vi "Read Browse Options.vi"(8 "error in (no error)":errorcluster, 11 "Path.lvclass in":refnum<class "Path.lvclass">) -> (0 "error out":errorcluster, 2 "BrowseOptions":T1, 3 "Path.lvclass out":refnum<class "Path.lvclass">)   [LabVIEW 2015, in "Path.lvclass"]
uses:
  Path.lvclass
  <vilib>/Utility/miscctls.llb/LVBrowseOptionsTypeDef.ctl
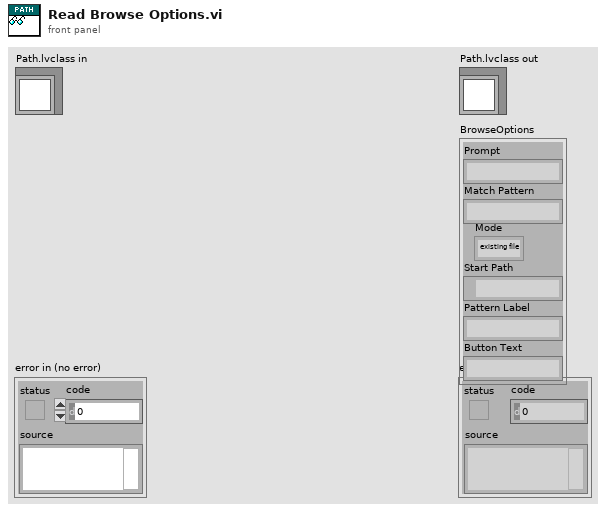
[diagram p1: front panel]
types:
  T1 = typedef "LVBrowseOptionsTypeDef.ctl" = cluster{"Prompt":string, "Match Pattern":string, "Mode":enum32{"existing file", "new file", "new or existing file", "existing dir", "new dir", "new or existing dir", "existing file (use LLBs)", "new file (use LLBs)", "new or existing file (use LLBs)", "new or existing file or directory (use LLBs)", "existing dir (use LLBs)", "new dir (use LLBs)", "new or existing dir (use LLBs)", "existing file or dir", "new file or dir", "new or existing file or dir", "existing file or dir (use LLBs)", "new file or dir (use LLBs)"}, "Start Path":path, "Pattern Label":string, "Button Text":string}
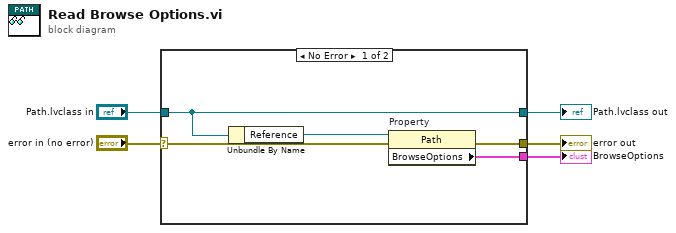
[diagram p0: block diagram]
diagram:
  n1 = case shown="No Error" "error in (no error)" {
    selector: "error in (no error)" -> [w6 w12]
    tunnel: [w9 w12] -> w4
    tunnel: [w8 w11] -> w2
    tunnel: "Path.lvclass in" -> [w8 w11]
    tunnel: [w10 _] -> w1
    frame No Error {
      n2 = Unbundle By Name(w8) -> ("Reference"=w7:refnum<vi>)
      n3 = property on="Property" class="Path"(reference=w7, error in=w6) -> (error out=w9:errorcluster, "BrowseOptions"=w10:T1)  [unwired: 1 out]
    }
    frame Error {
    }
  }
  "error out" <- w4
  "Path.lvclass out" <- w2
  "BrowseOptions" <- w1
